vi "Create User Events.vi"(8 "error in (no error)":errorcluster) -> (0 "error out":errorcluster, 3 "User Events":T1)   [LabVIEW 2020, in "User Events.lvlib"]
doc: "Create a boolean user event that will be used to stop the event loop from the message handling loop."
uses:
  User Events.lvlib
  controls/User Events ---typedef.ctl
  controls/Wake HL ---argument.ctl
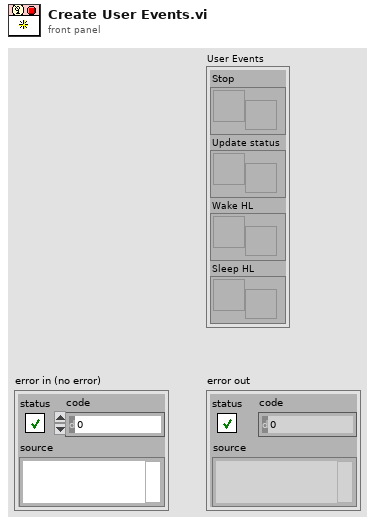
[diagram p1: front panel]
types:
  T1 = typedef "User Events ---typedef.ctl" = cluster{"Stop":refnum<user-event>, "Update status":refnum<user-event>, "Wake HL":refnum<user-event>, "Sleep HL":refnum<user-event>}
  T2 = typedef "Wake HL ---argument.ctl" = cluster{"Timeout":i32, "Module ID":i32, "Angle M1":i32, "Angle M2":i32}
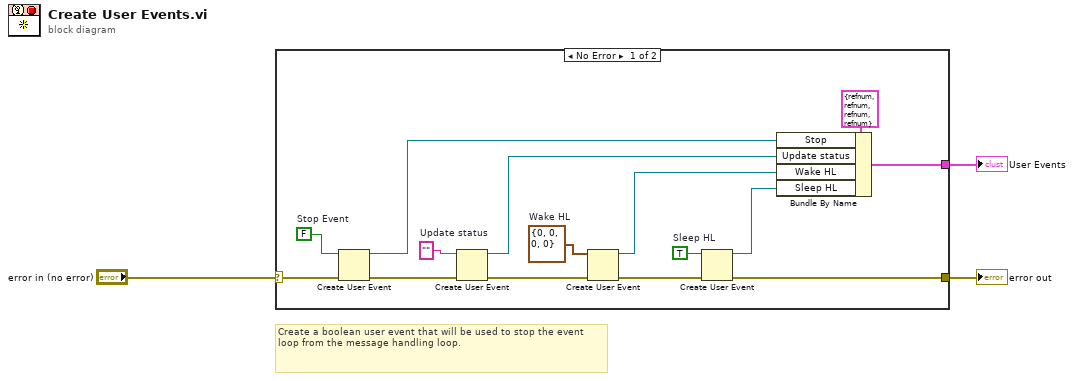
[diagram p0: block diagram]
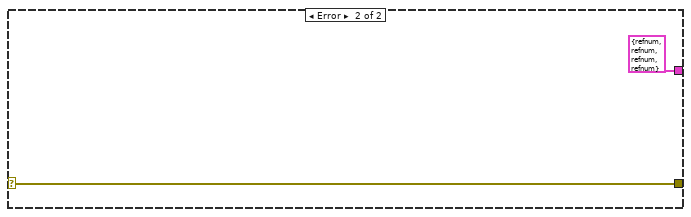
[diagram p2: hidden frame]
diagram:
  # "Create a boolean user event that will be used to stop the event loop from the message handling loop."
  n1 = case shown="No Error" "error in (no error)" {
    selector: "error in (no error)" -> [w17 w20]
    tunnel: [w6 w20] -> w3
    tunnel: [w11 T1 {"Stop"=refnum, "Update status"=refnum, "Wake HL"=refnum, "Sleep HL"=refnum} ("User Events")] -> w1
    frame No Error {
      w5 = TRUE  # Sleep HL
      w9 = T2 {"Timeout"=0, "Module ID"=0, "Angle M1"=0, "Angle M2"=0}  # Wake HL
      w15 = ""  # Update status
      w18 = FALSE  # Stop Event
      n2 = Create User Event(user event datatype=w18, error in=w17) -> (user event=w13:refnum<user-event>, error out=w16:errorcluster)
      n3 = Create User Event(user event datatype=w15, error in=w16) -> (user event=w12:refnum<user-event>, error out=w10:errorcluster)
      n4 = Create User Event(user event datatype=w9, error in=w10) -> (user event=w8:refnum<user-event>, error out=w7:errorcluster)
      n5 = Create User Event(user event datatype=w5, error in=w7) -> (user event=w4:refnum<user-event>, error out=w6:errorcluster)
      n6 = Bundle By Name(cluster=T1 {"Stop"=refnum, "Update status"=refnum, "Wake HL"=refnum, "Sleep HL"=refnum} ("User Events"), "Stop"=w13, "Update status"=w12, "Wake HL"=w8, "Sleep HL"=w4) -> (w11:T1)
    }
    frame Error {
    }
  }
  "error out" <- w3
  "User Events" <- w1
